vi "test_Build Queue Data.vi"(8 "error in (no error)":errorcluster, 11 "Data from FIFO":u64[](array[numeric])) -> (0 "error out":errorcluster, 3 "Data to Queue":T1[](array[typedef]))   [LabVIEW 2016]
uses:
  Host/Typedefs/Monitor Data Element.ctl
  Host/Typedefs/Monitor Data Operation.ctl
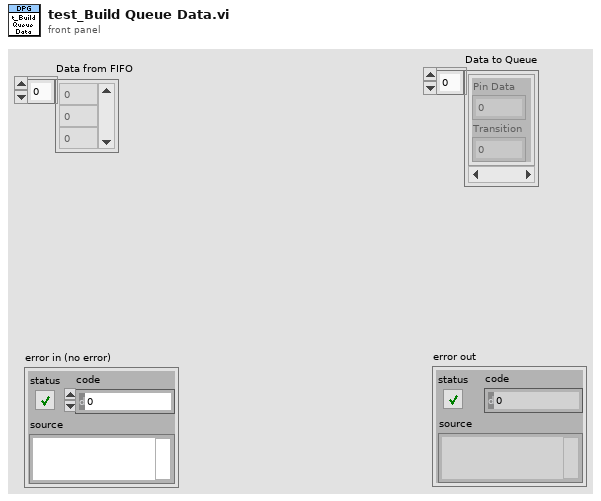
[diagram p1: front panel]
types:
  T1 = typedef "Monitor Data Element.ctl" = cluster{"Pin Data":u32, "Transition ":u32}
  T2 = typedef "Monitor Data Operation.ctl" = enum16{"Obtain", "Enqueue", "Read Elements", "Flush", "Release", "Read Last Element"}
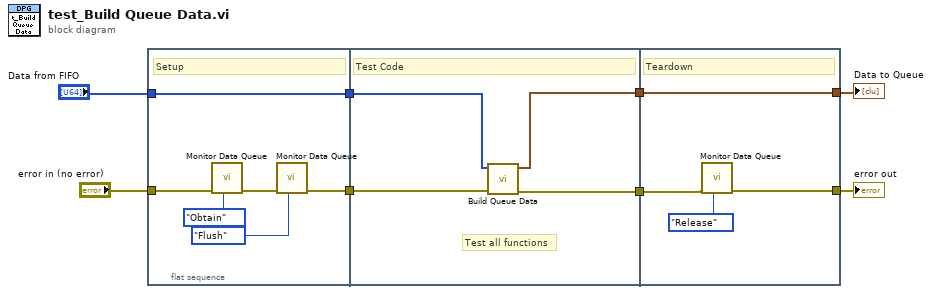
[diagram p0: block diagram]
diagram:
  n1 = flat-sequence {
    tunnel: "error in (no error)" -> [w13]
    tunnel: "Data from FIFO" -> [w14]
    tunnel: [w14] -> w6
    tunnel: [w9] -> w5
    tunnel: w6 -> [w17]
    tunnel: w5 -> [w18]
    tunnel: [w16] -> w3
    tunnel: [w15] -> w1
    tunnel: [w20] -> w7
    tunnel: w3 -> [w21]
    tunnel: [w22] -> w2
    tunnel: w1 -> [w22]
    frame #0 {
      # "Setup"
      n2 = call "Monitor Data Queue.vi"("Queue Function"=Monitor_Data_Operation."Obtain", "error in (no error)"=w13) -> ("error out"=w11:errorcluster)  [unwired: 6 in, 3 out]
      n3 = call "Monitor Data Queue.vi"("Queue Function"=Monitor_Data_Operation."Flush", "error in (no error)"=w11) -> ("error out"=w9:errorcluster)  [unwired: 6 in, 3 out]
    }
    frame #1 {
      # "Test all functions"
      # "Test Code"
      n4 = call "Build Queue Data.vi"("error in (no error)"=w18, "Data from FIFO"=w17) -> ("error out"=w16:errorcluster, "Data to Queue"=w15:T1[])  [unwired: 8 in]
    }
    frame #2 {
      # "Teardown"
      n5 = call "Monitor Data Queue.vi"("Queue Function"=Monitor_Data_Operation."Release", "error in (no error)"=w21) -> ("error out"=w20:errorcluster)  [unwired: 6 in, 3 out]
    }
  }
  "error out" <- w7
  "Data to Queue" <- w2
